vi "Qualisys_Dropped_Frames_Test.vi"(8 "error in (no error)":errorcluster) -> (0 "error out":errorcluster)   [LabVIEW 2019]
uses:
  Sub-VIs/System Message.ctl
  Sub-VIs/Enum_FileNewInterval.ctl
  Sub-VIs/RT Globals RD v1.0.vi
  <vilib>/ptbypt/NI_PtbyPt.lvlib
  Sub-VIs/FPGA Timekeeper 1.1b0/FPGA Timekeeper.lvlib
panel:
  out "Failed Init":bool
  out "error out 3":errorcluster
  in  "File save location":string="/home/lvuser/Qualisys"
  in  "stop":bool
  out "Resets":i32
  out "error out 2":errorcluster
  out "return 2":string
  out "length":i32
  out "Sample dt (us)":dbl format="%0.2f"
  out "return":i32
  out "ipAddress":string
  out "qtmPort":i32
  in  "ipAddress":string="10.10.59.100"
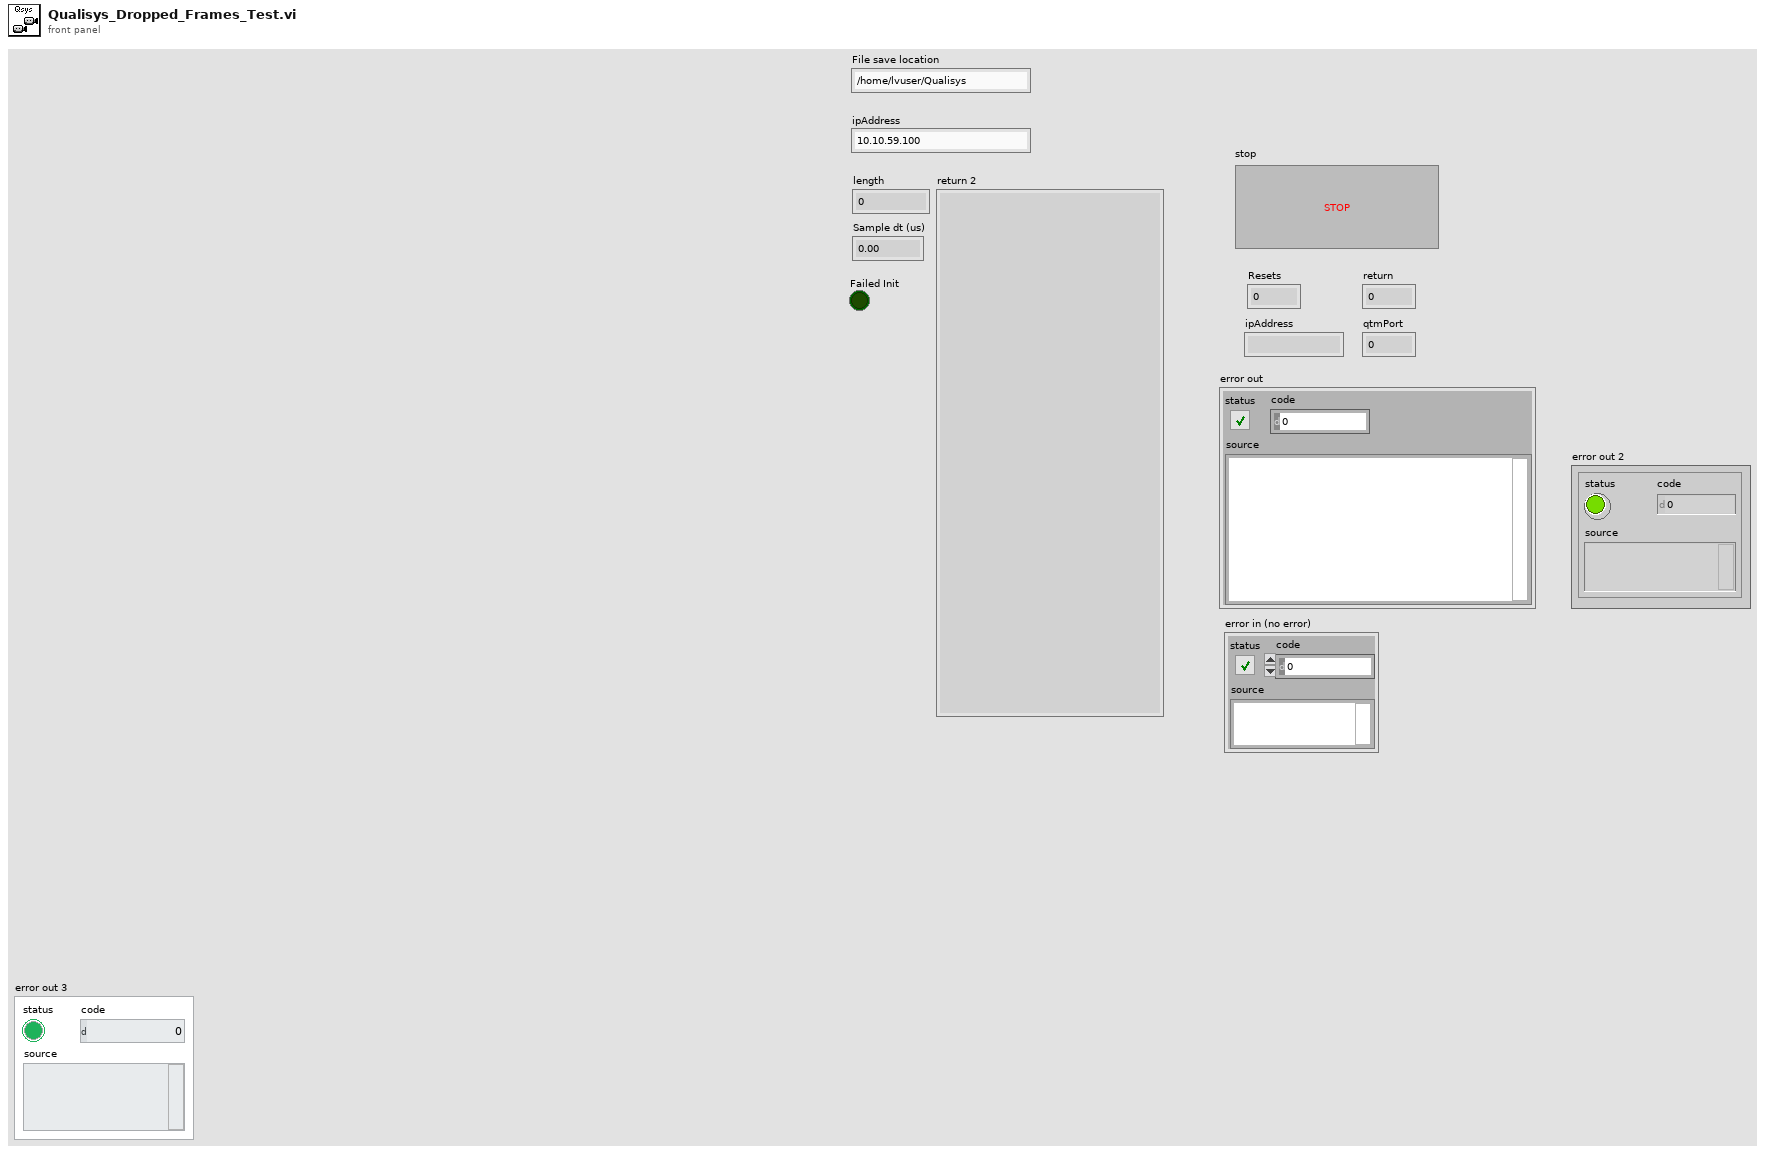
[diagram p1: front panel]
types:
  T1 = typedef "System Message.ctl" = cluster{"Message Tag":string, "Message Body":string, "Snooze Time (s)":dbl, "Snooze Alert?":bool, "Log Event?":bool, "Send Email":i32}
  T2 = enum16{"open", "replace", "create", "open or create", "replace or create", "replace or create with confirmation"}
  T3 = typedef "Enum_FileNewInterval.ctl" = enum16{"10 Min", "Hourly", "Daily", "Weekly", "Monthly"}
  T4 = typedef "LVDateTimeRec.ctl" = cluster{"fractional second":dbl, "second":i32, "minute":i32, "hour":i32, "day of month":i32, "month":i32, "year":i32, "day of week":i32, "day of year":i32, "DST":i32}
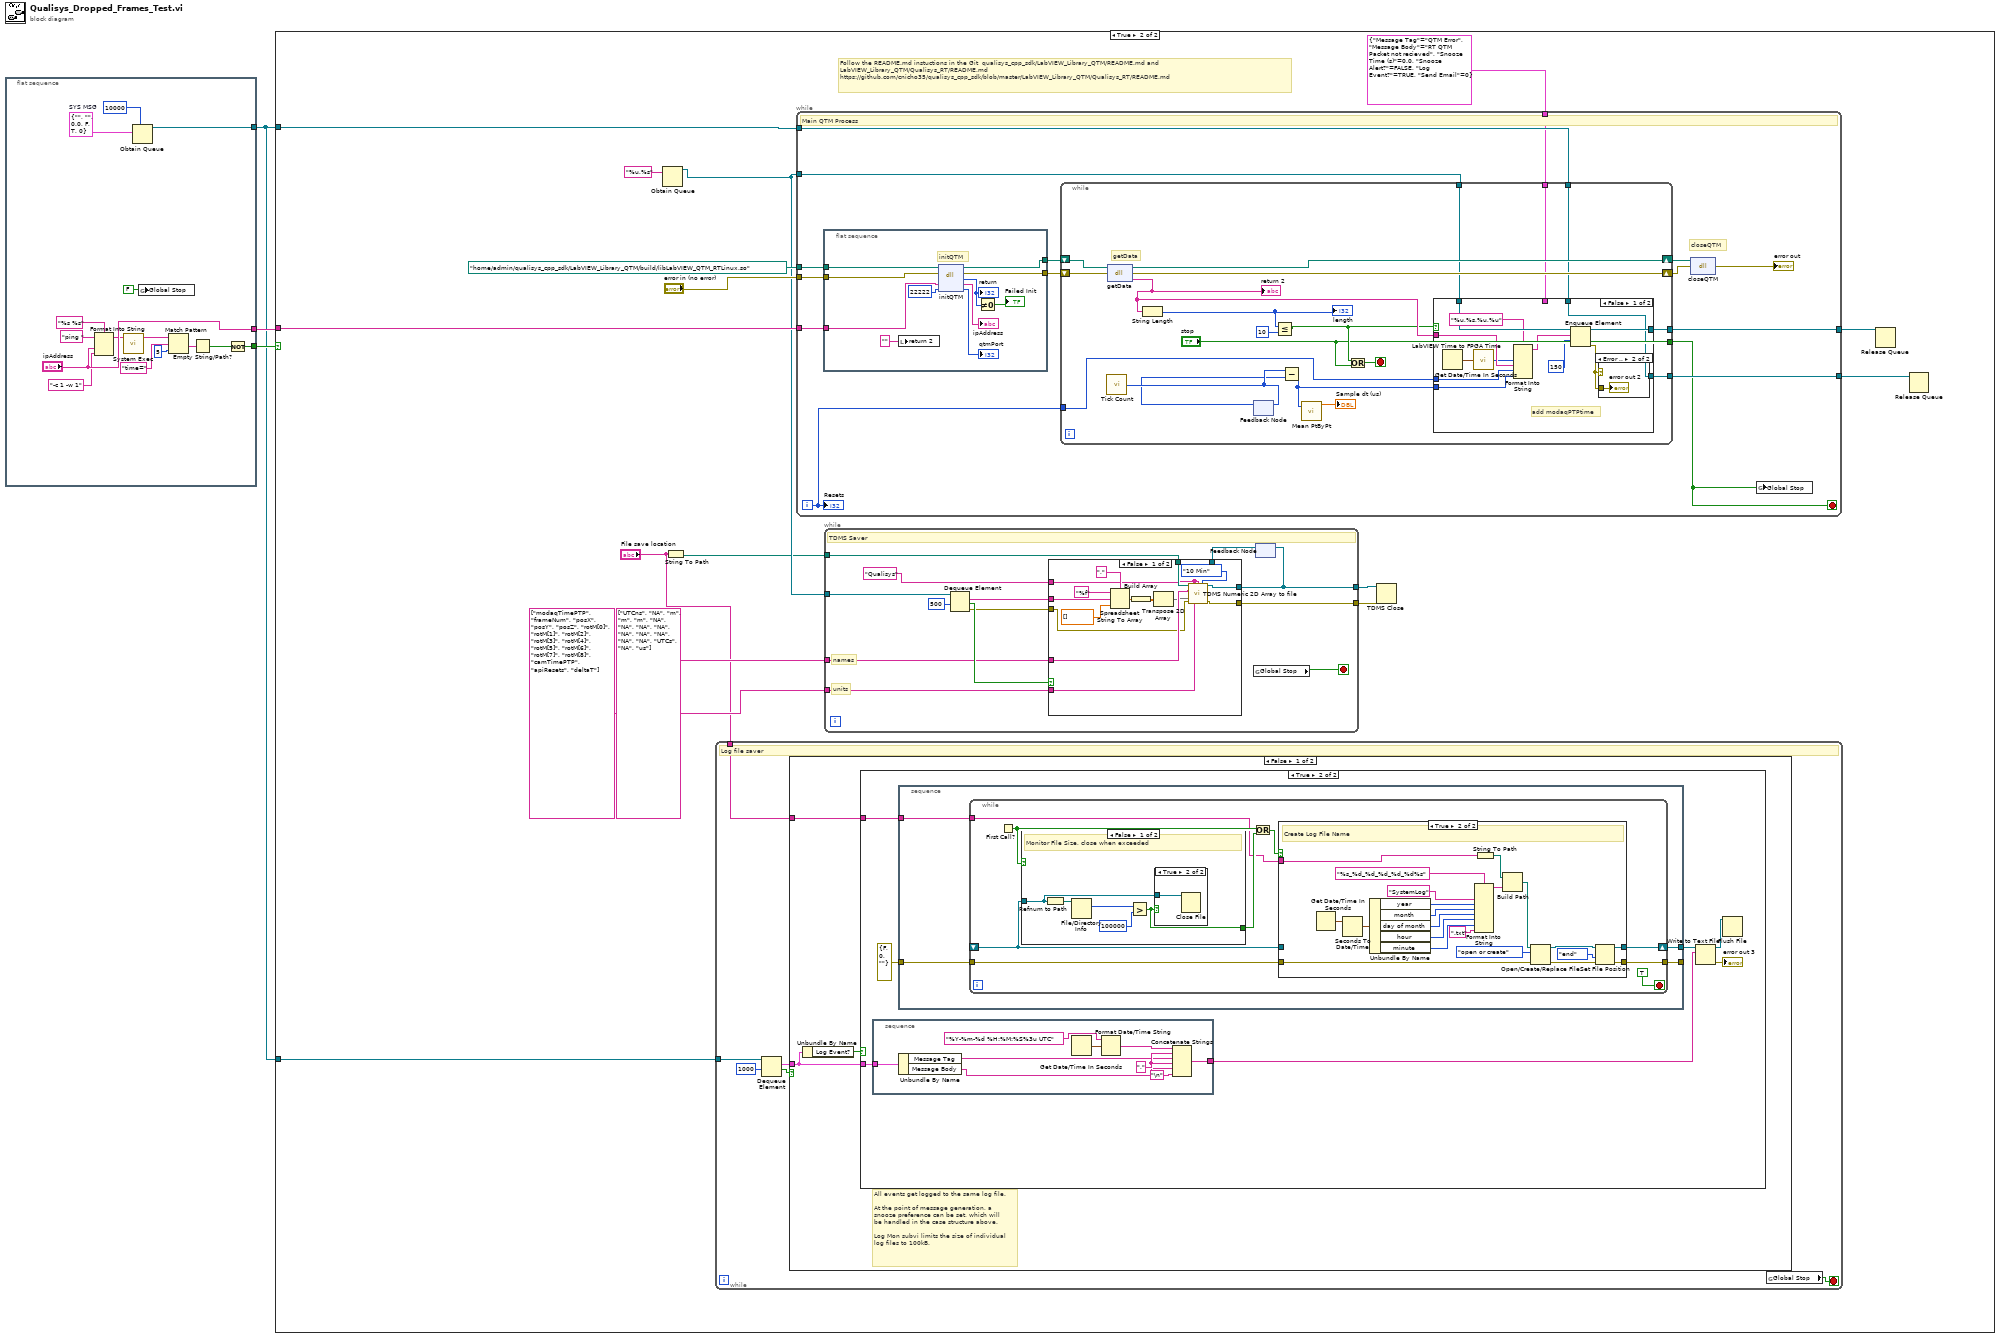
[diagram p0: block diagram]
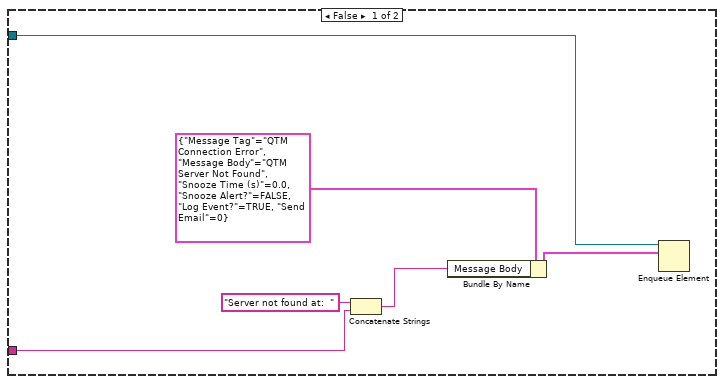
[diagram p2: hidden frame]
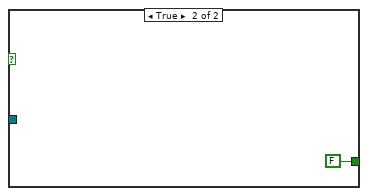
[diagram p5: hidden frame]
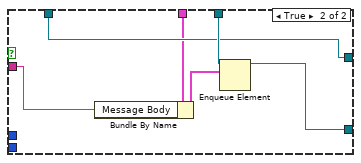
[diagram p10: hidden frame]
diagram:
  n1 = flat-sequence {
    tunnel: ["ipAddress"] -> w3
    tunnel: [w8] -> w2
    tunnel: [w6] -> w1
    frame #0 {
      w7 = T1 {"Message Tag"="", "Message Body"="", "Snooze Time (s)"=0.0, "Snooze Alert?"=FALSE, "Log Event?"=TRUE, "Send Email"=0}  # SYS MSG
      n2 = Format Into String(format string="%s %s", initial string="ping ", "ipAddress", "-c 1 -w 1" ("input 2")) -> (resulting string=w14:string)  [unwired: 1 in, 1 out]
      n3 = call <vilib>:"System Exec.vi"("command line"=w14) -> ("standard output"=w13:string)  [unwired: 7 in, 3 out]
      n4 = Obtain Queue(max queue size (-1, unlimited)=10000, element data type=w7) -> (queue out=w6:refnum<queue>)  [unwired: 3 in, 2 out]
      n5 = global write "RT Globals RD v1.0.vi" "Global Stop"(FALSE ("Global Stop")) -> ()
      n6 = Match Pattern(string=w13, regular expression="time=" ("search string"), offset (0)=5) -> (after substring=w10:string)  [unwired: 3 out]
      n7 = Empty String/Path?(string/path=w10) -> (empty?=w9:bool)
      n8 = Not(x=w9) -> (.not. x?=w8:bool)
    }
  }
  n9 = case shown="True" w2 {
    tunnel: w3 -> [w19 w38]
    tunnel: w1 -> [w24 w37]
    tunnel: w1 -> [_ w26]
    frame False {
      n10 = Concatenate Strings("Server not found at:  " ("Message Body"), w19) -> (w20:string)
      n11 = Bundle By Name(cluster=T1 {"Message Tag"="QTM Connection Error", "Message Body"="QTM Server Not Found", "Snooze Time (s)"=0.0, "Snooze Alert?"=FALSE, "Log Event?"=TRUE, "Send Email"=0} ("element"), "Message Body"=w20) -> (w22:T1)
      n12 = Enqueue Element(queue=w24, element=w22) -> ()  [unwired: 2 in, 3 out]
    }
    frame True {
      # "Follow the README.md instuctions in the Git  qualisys_cpp_sdk/LabVIEW_Library_QTM/README.md and\nLabVIEW_Library_QTM/Qualisys_RT/README.md\nhttps://github.com/cnicho35/qualisys_cpp_sdk/blob/master/LabVIEW_Library_QTM/Qualisys_RT/README.md"
      n13 = Obtain Queue(element data type="%u,%s" ("format string")) -> (queue out=w32:refnum<queue>)  [unwired: 4 in, 2 out]
      n14 = String To Path(string="File save location") -> (path=w27:path)
      n15 = while {
        tunnel: w26 -> [w43]
        tunnel: "File save location" -> [w41]
        stop <- w42 stop-if-true
        # "Log file saver"
        n16 = Dequeue Element(queue=w43, timeout in ms (-1)=1000) -> (element=w46:T1, timed out?=w45:bool)  [unwired: 1 in, 2 out]
        n17 = case shown="False" w45 {
          tunnel: w46 -> [w49 _]
          tunnel: w41 -> [w47 _]
          frame False {
            # "All events get logged to the same log file. \n\nAt the point of message generation, a \nsnooze preference can be set, which will\nbe handled in the case structure above.\n\nLog Mon subvi limits the size of individual\nlog files to 100kB."
            n18 = Unbundle By Name(w49) -> ("Log Event?"=w48:bool)
            n19 = case shown="True" w48 {
              tunnel: w49 -> [_ w55]
              tunnel: w47 -> [_ w50]
              frame False {
              }
              frame True {
                n20 = stacked-sequence {
                  tunnel: [w105] -> w54
                  tunnel: w55 -> [w102]
                  frame #0 {
                    w106 = ","
                    n21 = Unbundle By Name(w102) -> ("Message Tag"=w103:string, "Message Body"=w104:string)
                    n22 = Get Date/Time In Seconds() -> (seconds since 1Jan1904=w108:timestamp)
                    n23 = Format Date/Time String(time format string (%c)="%Y-%m-%d %H:%M:%S%3u UTC", seconds (now)=w108) -> (date/time string=w101:string)  [unwired: 1 in]
                    n24 = Concatenate Strings(w101, w106, w103, w106, w104, "\n") -> (w105:string)
                  }
                }
                n25 = stacked-sequence {
                  tunnel: [w59] -> _
                  tunnel: [w60] -> w53
                  tunnel: errorcluster {"status"=FALSE, "code"=0, "source"=""} ("error in") -> [w58]
                  tunnel: w50 -> [w57]
                  frame #0 {
                    n26 = while {
                      tunnel: w58 -> [w69]
                      tunnel: [w68] -> w59
                      shift-right: [w66] -> w60
                      shift-left: _ -> [w65]
                      tunnel: w57 -> [w61]
                      stop <- TRUE stop-if-true
                      n27 = First Call?() -> (First Call?: T/F=w63:bool)
                      n28 = case shown="False" w63 {
                        tunnel: w65 -> [w71 _]
                        tunnel: [w70 FALSE] -> w62
                        frame False {
                          # "Monitor File Size, close when exceeded"
                          n29 = Refnum to Path(1:w71) -> (0:w74:path)
                          n30 = File/Directory Info(path=w74) -> (size=w73:i64)  [unwired: 1 in, 6 out]
                          n31 = Greater?(x=w73, y=i64 100000) -> (0:w70:bool)
                          n32 = case shown="True" w70 {
                            tunnel: w71 -> [_ w75]
                            frame False {
                            }
                            frame True {
                              n33 = Close File(refnum=w75) -> ()  [unwired: 1 in, 2 out]
                            }
                          }
                        }
                        frame True {
                        }
                      }
                      n34 = Or(x=w63, y=w62) -> (x .or. y?=w64:bool)
                      n35 = case shown="True" w64 {
                        tunnel: w69 -> [w77 w85]
                        tunnel: [w77 w83] -> w68
                        tunnel: [w78 w81] -> w66
                        tunnel: w65 -> [w78 _]
                        tunnel: w61 -> [_ w79]
                        frame False {
                        }
                        frame True {
                          # "Create Log File Name"
                          n36 = Get Date/Time In Seconds() -> (seconds since 1Jan1904=w86:timestamp)
                          n37 = Seconds To Date/Time(time stamp (now)=w86) -> (date time rec=w99:T4)  [unwired: 1 in]
                          n38 = Unbundle By Name(w99) -> ("year"=w92:i32, "month"=w91:i32, "day of month"=w90:i32, "hour"=w89:i32, "minute"=w88:i32)
                          n39 = Format Into String(format string="%s_%d_%d_%d_%d_%d%s", "SystemLog" ("name or relative path"), w92, w91, w90, w89, w88, ".txt" ("name or relative path")) -> (resulting string=w87:string)  [unwired: 2 in, 1 out]
                          n40 = String To Path(string=w79) -> (path=w82:path)
                          n41 = Build Path(base path=w82, name or relative path=w87) -> (appended path=w93:path)
                          n42 = Open/Create/Replace File(file path (use dialog)=w93, error in=w85, operation (0:open)=T2."open or create") -> (refnum out=w80:refnum<file>, error out=w84:errorcluster)  [unwired: 3 in, 1 out]
                          n43 = Set File Position(refnum=w80, from (0:start)=enum16{"start", "end", "current"}."end", error in=w84) -> (refnum out=w81:refnum<file>, error out=w83:errorcluster)  [unwired: 1 in]
                        }
                      }
                    }
                  }
                }
                n44 = Write to Text File(file (use dialog)=w53, text=w54) -> (refnum out=w56:refnum<file>, error out=→"error out 3":errorcluster)  [unwired: 2 in, 1 out]
                n45 = Flush File(refnum=w56) -> ()  [unwired: 1 in, 2 out]
              }
            }
          }
          frame True {
          }
        }
        n46 = global read "RT Globals RD v1.0.vi" "Global Stop"() -> (w42:bool)
      }
      n47 = while {
        tunnel: "error in (no error)" -> [w148]
        tunnel: w32 -> [w147]
        tunnel: w37 -> [w146]
        tunnel: path "/home/admin/qualisys_cpp_sdk/LabVIEW_Library_QTM/build/libLabVIEW_QTM_RTLinux.so" ("path in") -> [w145]
        tunnel: w38 -> [w144]
        tunnel: [w143] -> w30
        tunnel: [w142] -> w29
        tunnel: T1 {"Message Tag"="QTM Error", "Message Body"="RT QTM Packet not recieved", "Snooze Time (s)"=0.0, "Snooze Alert?"=FALSE, "Log Event?"=TRUE, "Send Email"=0} ("element") -> [w141]
        i -> [w139]
        stop <- w140 stop-if-true
        # "closeQTM"
        # "Main QTM Process"
        n48 = flat-sequence {
          tunnel: [w203] -> w153
          tunnel: [w202] -> w151
          tunnel: w148 -> [w200]
          tunnel: w145 -> [w199]
          tunnel: w144 -> [w198]
          frame #0 {
            # "initQTM"
            n49 = local write "return 2"("") -> ()
            n50 = dll-call lib="home/admin/qualisys_cpp_sdk/LabVIEW_Library_QTM/build/libLabVIEW_QTM_RTLinux.so" fn="initQTM"(path in=w199, error in=w200, "ipAddress"=w198, "qtmPort"=22222) -> (path out=w203:path, error out=w202:errorcluster, "return"=w194:i32, "ipAddress"=→"ipAddress":string, "qtmPort"=→"qtmPort":i32)  [unwired: 1 in]
            "return" <- w194
            n51 = Not Equal To 0?(x=w194) -> (x != 0?=→"Failed Init":bool)
          }
        }
        n52 = while {
          shift-right: [w172] -> w152
          shift-left: w153 -> [w173]
          shift-right: [w170] -> w150
          shift-left: w151 -> [w171]
          tunnel: ["stop"] -> w140
          tunnel: w147 -> [w166]
          tunnel: w146 -> [w165]
          tunnel: [w163] -> w143
          tunnel: [w162] -> w142
          tunnel: w141 -> [w158]
          tunnel: w139 -> [w156]
          stop <- w167 stop-if-true
          # "getData"
          n53 = call "Tick Count"() -> ("Tick Count(uSec)"=w169:u32)
          n54 = dll-call lib="home/admin/qualisys_cpp_sdk/LabVIEW_Library_QTM/build/libLabVIEW_QTM_RTLinux.so" fn="getData"(path in=w173, error in=w171) -> (path out=w172:path, error out=w170:errorcluster, "return"=w164:string)  [unwired: 1 in]
          "return 2" <- w164
          n55 = String Length(string=w164) -> (length=w161:i32)
          "length" <- w161
          n56 = feedback-in #1(w169) -> ()
          n57 = feedback #1() -> (w168:u32)  [unwired: 1 in]
          n58 = Less Or Equal?(x=w161, y=10) -> (x <= y?=w159:bool)
          n59 = Subtract(x=w169, y=w168) -> (x-y=w154:u32)
          n60 = call <vilib>:"Mean PtByPt.vi"("x"=w154) -> ("mean"=→"Sample dt (us)":dbl)  [unwired: 3 in, 1 out]
          n61 = Or(x=w159, y="stop") -> (x .or. y?=w167:bool)
          n62 = case shown="False" w159 {
            tunnel: w166 -> [w185 w190]
            tunnel: w164 -> [w181 w188]
            tunnel: w165 -> [w176 w192]
            tunnel: [w177 w190] -> w163
            tunnel: [w176 w191] -> w162
            tunnel: w158 -> [_ w187]
            tunnel: w156 -> [w175 _]
            tunnel: w154 -> [w174 _]
            frame False {
              # "add modaqPTPtime"
              n63 = Get Date/Time In Seconds() -> (seconds since 1Jan1904=w179:timestamp)
              n64 = call "LabVIEW Time to FPGA Time.vi"("LabVIEW time"=w179) -> ("FPGA time (ns)"=w178:u64)
              n65 = Format Into String(format string="%u,%s,%u,%u", w178, w181, w175, w174) -> (resulting string=w182:string)  [unwired: 2 in, 1 out]
              n66 = Enqueue Element(queue=w185, element=w182, timeout in ms (-1)=150) -> (queue out=w177:refnum<queue>, error out=w180:errorcluster)  [unwired: 1 in, 1 out]
              n67 = case shown="Error .." w180 {
                tunnel: w180 -> [_ w186]
                frame No Error {
                }
                frame Error {
                  "error out 2" <- w186
                }
              }
            }
            frame True {
              n68 = Bundle By Name(cluster=w187, "Message Body"=w188) -> (w189:T1)
              n69 = Enqueue Element(queue=w192, element=w189) -> (queue out=w191:refnum<queue>)  [unwired: 2 in, 2 out]
            }
          }
        }
        n70 = dll-call lib="home/admin/qualisys_cpp_sdk/LabVIEW_Library_QTM/build/libLabVIEW_QTM_RTLinux.so" fn="closeQTM"(path in=w152, error in=w150) -> (error out=→"error out":errorcluster)  [unwired: 2 in, 1 out]
        n71 = global write "RT Globals RD v1.0.vi" "Global Stop"(w140) -> ()
        "Resets" <- w139
      }
      n72 = while {
        tunnel: w32 -> [w121]
        tunnel: w27 -> [w116]
        tunnel: string[] ["modaqTimePTP", "frameNum", "posX", "posY", "posZ", "rotM[0]", "rotM[1]", "rotM[2]", "rotM[3]", "rotM[4]", "rotM[5]", "rotM[6]", "rotM[7]", "rotM[8]", "camTimePTP", "apiResets", "deltaT"] ("Channel Names") -> [w115]
        tunnel: string[] ["UTCns", "NA", "m", "m", "m", "NA", "NA", "NA", "NA", "NA", "NA", "NA", "NA", "NA", "UTCs", "NA", "us"] ("Channel Names") -> [w114]
        tunnel: [w112] -> w34
        tunnel: [w113] -> w33
        stop <- w117 stop-if-true
        # "units"
        # "names"
        # "TDMS Saver"
        n73 = Dequeue Element(queue=w121, timeout in ms (-1)=500) -> (element=w118:string, timed out?=w119:bool, error out=w110:errorcluster)  [unwired: 1 in, 1 out]
        n74 = global read "RT Globals RD v1.0.vi" "Global Stop"() -> (w117:bool)
        n75 = feedback #2() -> (w111:refnum<k34>)  [unwired: 1 in]
        n76 = case shown="False" w119 {
          tunnel: w118 -> [w136 _]
          tunnel: w116 -> [w131 _]
          tunnel: "Qualisys" ("name or relative path") -> [w129 _]
          tunnel: w115 -> [w133 _]
          tunnel: w114 -> [w132 _]
          tunnel: [w130 w138] -> w112
          tunnel: [w126 w137] -> w113
          tunnel: w111 -> [_ w138]
          tunnel: w110 -> [w127 w137]
          frame False {
            n77 = Spreadsheet String To Array(delimiter (Tab)=",", format string="%f", spreadsheet string=w136, array type (2D Dbl)=dbl[] []) -> (array=w125:dbl[])
            n78 = Build Array(w125) -> (w124:dbl[][])
            n79 = Transpose 2D Array(2D array=w124) -> (transposed array=w122:dbl[][])
            n80 = call "TDMS Numeric 2D Array to file.vi"("Base path"=w131, "Group Name"=w129, "FileName"=w129, "Interval"=Enum_FileNewInterval."10 Min", "Channel Names"=w133, "2D array"=w122, "error in (no error)"=w127, "Channel Units"=w132) -> ("file out"=w130:refnum<k34>, "error out"=w126:errorcluster)  [unwired: 6 in]
          }
          frame True {
          }
        }
        n81 = feedback-in #2(w112) -> ()
      }
      n82 = TDMS Close(8:w33, 11:w34) -> ()  [unwired: 2 out]
      n83 = Release Queue(queue=w30) -> ()  [unwired: 2 in, 3 out]
      n84 = Release Queue(queue=w29) -> ()  [unwired: 2 in, 3 out]
    }
  }
